vi "Write Coords.vi"(8 "error in":errorcluster, 9 "Index":i32, 10 "Adr":string, 11 "XLS in":refnum<class "XLS.lvclass">) -> (0 "error out":errorcluster, 3 "XLS out":refnum<class "XLS.lvclass">)   [LabVIEW 2017, in "Report_lib.lvlib" / "XLS.lvclass"]
doc: "Set Excel coordinates\nin necessary format"
uses:
  XLS.lvclass
  XLS.lvclass/XLS.ctl
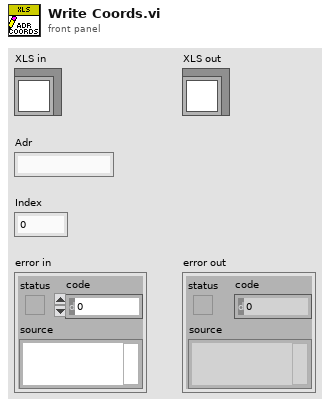
[diagram p1: front panel]
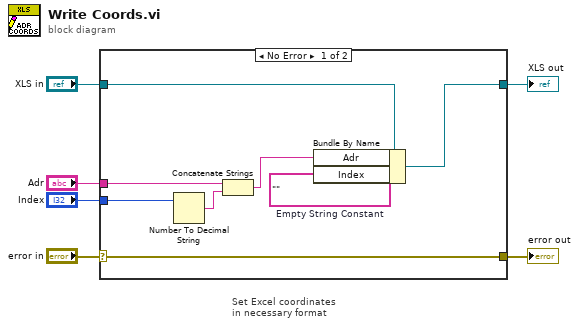
[diagram p0: block diagram]
diagram:
  # "Set Excel coordinates\nin necessary format"
  n1 = case shown="No Error" "error in" {
    selector: "error in" -> [w14 w15]
    tunnel: [w14 w15] -> w5
    tunnel: [w12 w16] -> w3
    tunnel: "XLS in" -> [w13 w16]
    tunnel: "Adr" -> [w10 _]
    tunnel: "Index" -> [w9 _]
    frame No Error {
      w8 = ""  # Empty String Constant
      n2 = Number To Decimal String(number=w9) -> (decimal integer string=w11:string)  [unwired: 1 in]
      n3 = Concatenate Strings(w10, w11) -> (w7:string)
      n4 = Bundle By Name(cluster=w13, "Adr"=w7, "Index"=w8) -> (w12:refnum<class "XLS.lvclass">)
    }
    frame Error {
    }
  }
  "error out" <- w5
  "XLS out" <- w3
